vi "Read Form Server Configuration.vi"(8 "error in (no error)":errorcluster, 11 "Form Server in":refnum<class "Form Server.lvclass">) -> (0 "error out":errorcluster, 2 "Form Server Configuration.lvlib:Form Server Configuration.lvclass":refnum<class "Form Server Configuration.lvclass">, 3 "Form Server out":refnum<class "Form Server.lvclass">)   [LabVIEW 2020, in "Form Server.lvlib" / "Form Server.lvclass"]
uses:
  Form Server.lvclass
  Form Server Configuration/Form Server Configuration.lvclass
  Form Server.lvclass/Form Server.ctl
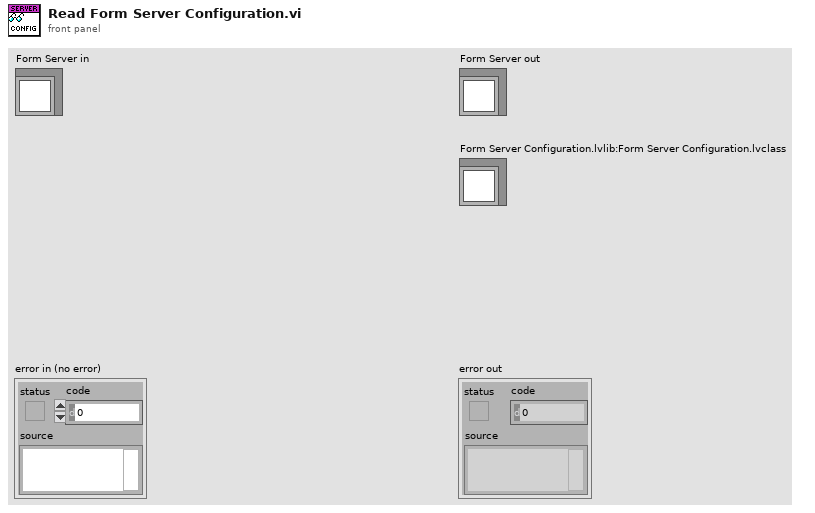
[diagram p1: front panel]
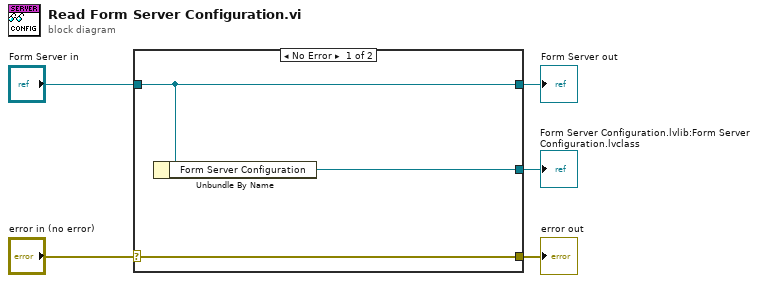
[diagram p0: block diagram]
diagram:
  n1 = case shown="No Error" "error in (no error)" {
    selector: "error in (no error)" -> [w8 w9]
    tunnel: [w8 w9] -> w4
    tunnel: [w7 w10] -> w2
    tunnel: "Form Server in" -> [w7 w10]
    tunnel: [w6 _] -> w1
    frame No Error {
      n2 = Unbundle By Name(w7) -> ("Form Server Configuration"=w6:refnum<class "Form Server Configuration.lvclass">)
    }
    frame Error {
    }
  }
  "error out" <- w4
  "Form Server out" <- w2
  "Form Server Configuration.lvlib:Form Server Configuration.lvclass" <- w1
